vi "GetStatus.vi"(6 "Stat Bin":refnum<vi>, 8 "error in (no error)":errorcluster, 11 "Rele in":refnum<class "Rele.lvclass">) -> (0 "error out":errorcluster, 2 "Status Int":i32, 3 "Rele out":refnum<class "Rele.lvclass">)   [LabVIEW 2012, in "Rele.lvclass"]
uses:
  Rele.lvclass
  Controlador.lvclass
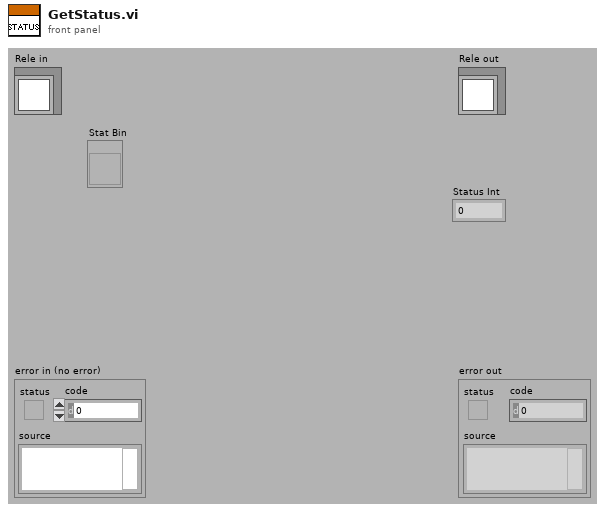
[diagram p1: front panel]
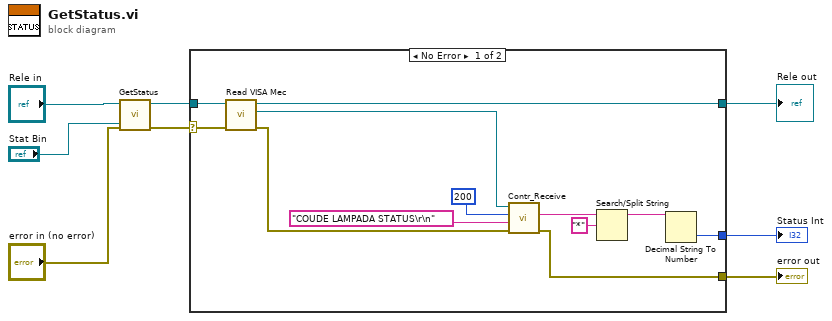
[diagram p0: block diagram]
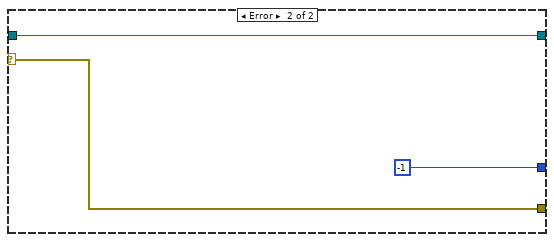
[diagram p2: hidden frame]
diagram:
  n1 = call-parent "GetStatus.vi"("Stat Bin"="Stat Bin", "error in (no error)"="error in (no error)", "Device in"="Rele in") -> ("error out"=w5:errorcluster, "Device out"=w4:refnum<class "Rele.lvclass">)  [unwired: 6 in, 1 out]
  n2 = case shown="No Error" w5 {
    selector: w5 -> [w10 w21]
    tunnel: w4 -> [w17 w22]
    tunnel: [w16 w22] -> w3
    tunnel: [w15 w21] -> w2
    tunnel: [w11 -1] -> w1
    frame No Error {
      n3 = call-dynamic "Read VISA Mec.vi"("error in (no error)"=w10, "Controlador in"=w17) -> ("error out"=w20:errorcluster, "VISA Mec"=w19:refnum<visa-resource-name>, "Controlador out"=w16:refnum<class "Rele.lvclass">)  [unwired: 7 in]
      n4 = call "Contr_Receive.vi"("error in"=w20, "Command to SIFS"="COUDE LAMPADA STATUS\r\n", "wait after tx"=u32 200, "VISA resource name"=w19) -> ("error out"=w15:errorcluster, "Response from SIFS"=w14:string)  [unwired: 2 out]
      n5 = Search/Split String(string=w14, search string/char (-)="*") -> (substring before match=w12:string)  [unwired: 1 in, 2 out]
      n6 = Decimal String To Number(string=w12) -> (number=w11:i32)  [unwired: 2 in, 1 out]
    }
    frame Error {
    }
  }
  "error out" <- w2
  "Rele out" <- w3
  "Status Int" <- w1
